vi "Generate Comments.vi"(7 "error in (no error)":errorcluster, 8 "Ring in":refnum<vi>, 9 "cluster":T1) -> (0 "error out":errorcluster, 2 "Comments":string)   [LabVIEW 2016, in "Transport.lvclass"]
uses:
  Transport.lvclass
  Typedefs/Comments-cluster.ctl
  <userlib>/LevyLab/Krohn Hite 7008/typedefs/Gain-Enum.ctl
  <userlib>/LevyLab/Krohn Hite 7008/typedefs/Shunt-Enum.ctl
  <userlib>/LevyLab/Krohn Hite 7008/KH7008.lvclass
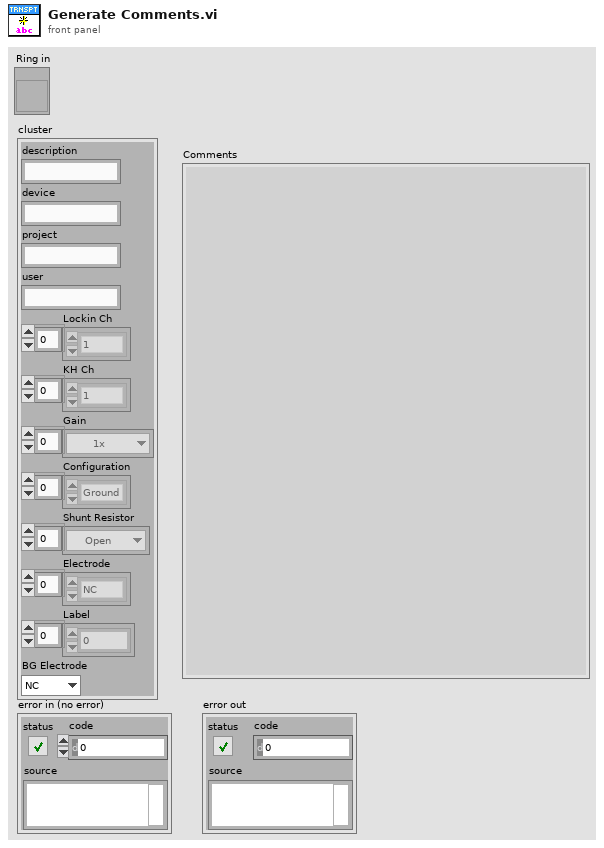
[diagram p1: front panel]
types:
  T1 = typedef "Transport.lvclass/Comments-cluster.ctl" = cluster{"description":string, "device":string, "project":string, "user":string, "Lockin Ch":enum16{"1", "2", "3", "4", "5", "6", "7", "8"}[], "KH Ch":enum16{"1", "2", "3", "4", "5", "6", "7", "8"}[], "Gain":T2[], "Configuration":enum16{"Ground", "Current", "Voltage", "Gate"}[], "Shunt Resistor":T3[], "Electrode":enum16{"NC", "26", "27", "28", "1", "2", "3", "4", "5", "6", "7", "8", "9", "10", "11", "12", "13", "14", "15", "16", "17", "18", "19", "20", "21", "22", "23", "24", "25"}[], "Label":u16[], "BG Electrode":enum16{"NC", "26", "27", "28", "1", "2", "3", "4", "5", "6", "7", "8", "9", "10", "11", "12", "13", "14", "15", "16", "17", "18", "19", "20", "21", "22", "23", "24", "25"}}
  T2 = typedef "KH7008.lvclass/Gain-Enum.ctl" = enum16{"1x", "10x", "100x", "1000x"}
  T3 = typedef "KH7008.lvclass/Shunt-Enum.ctl" = enum16{"Open", "50 Ohms", "500 Ohms", "5k Ohms", "50k Ohms"}
  T4 = enum16{"NC", "26", "27", "28", "1", "2", "3", "4", "5", "6", "7", "8", "9", "10", "11", "12", "13", "14", "15", "16", "17", "18", "19", "20", "21", "22", "23", "24", "25"}[]
  T5 = enum16{"NC", "26", "27", "28", "1", "2", "3", "4", "5", "6", "7", "8", "9", "10", "11", "12", "13", "14", "15", "16", "17", "18", "19", "20", "21", "22", "23", "24", "25"}
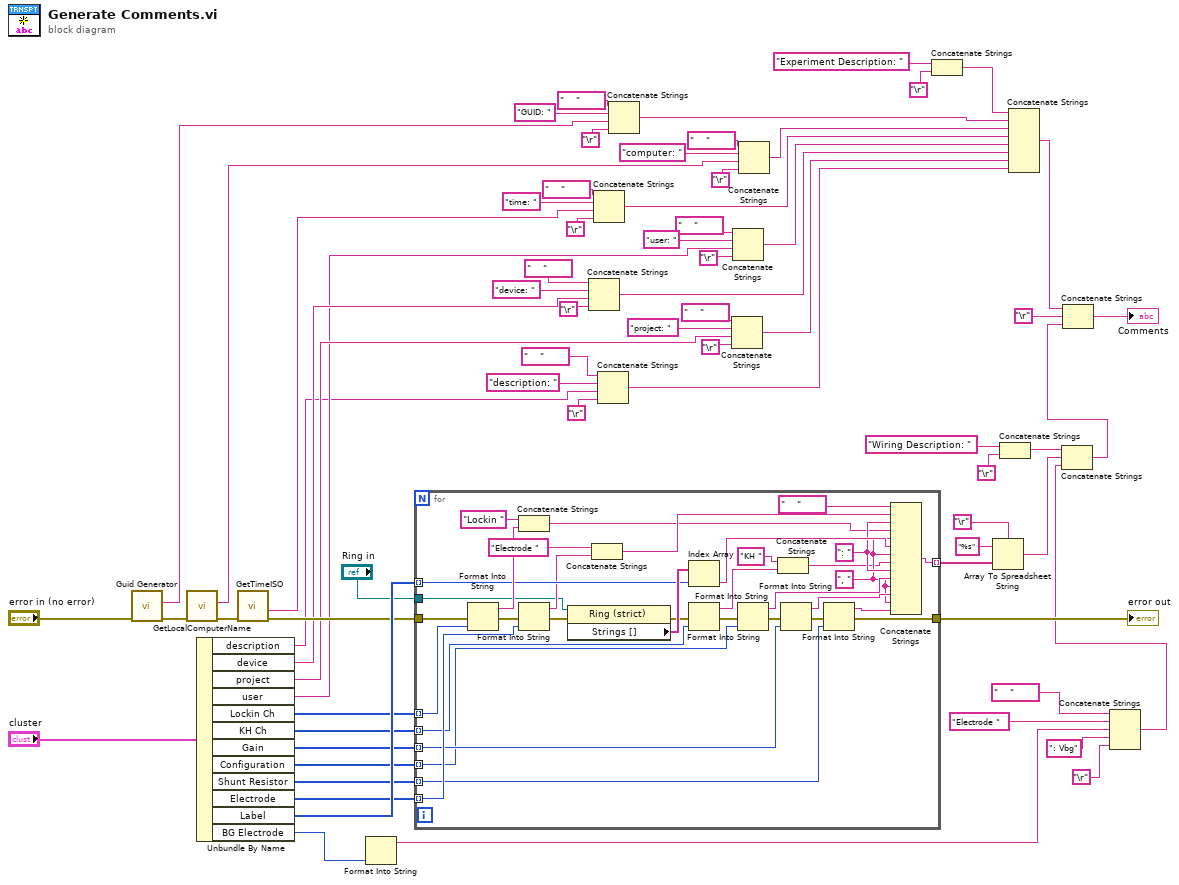
[diagram p0: block diagram]
diagram:
  n1 = call <vilib>:"Guid Generator.vi"("error in (no error)"="error in (no error)") -> ("error out"=w42:errorcluster, "GUID"=w26:string)  [unwired: 9 in]
  n2 = call <userlib>:"GetLocalComputerName.vi"("error in (no error)"=w42) -> ("error out"=w38:errorcluster, "Name"=w22:string)  [unwired: 9 in]
  n3 = Unbundle By Name("cluster") -> ("description"=w40:string, "device"=w50:string, "project"=w49:string, "user"=w48:string, "Lockin Ch"=w64:enum16{"1", "2", "3", "4", "5", "6", "7", "8"}[], "KH Ch"=w65:enum16{"1", "2", "3", "4", "5", "6", "7", "8"}[], "Gain"=w66:T2[], "Configuration"=w67:enum16{"Ground", "Current", "Voltage", "Gate"}[], "Shunt Resistor"=w68:T3[], "Electrode"=w69:T4, "Label"=w70:u16[], "BG Electrode"=w7:T5)
  n4 = call "GetTimeISO.vi"("error in (no error)"=w38) -> ("error out"=w58:errorcluster, "ISO 8601 date-time string"=w41:string)  [unwired: 8 in, 1 out]
  n5 = Format Into String(w7) -> (resulting string=w5:string)  [unwired: 3 in, 1 out]
  n6 = for {
    tunnel: w64 -> [w104] mode=indexing
    tunnel: w65 -> [w83] mode=indexing
    tunnel: w66 -> [w94] mode=indexing
    tunnel: w67 -> [w92] mode=indexing
    tunnel: w68 -> [w87] mode=indexing
    tunnel: w69 -> [w96] mode=indexing
    tunnel: w70 -> [w98] mode=indexing
    tunnel: [w100] -> w59 mode=indexing
    tunnel: "Ring in" -> [w82]
    tunnel: w58 -> [w81]
    tunnel: [w74] -> w57
    w89 = ", "
    w93 = ": "
    n7 = Format Into String(error in=w81, w104) -> (resulting string=w102:string, error out=w80:errorcluster)  [unwired: 2 in]
    n8 = Concatenate Strings("Lockin ", w102) -> (w71:string)
    n9 = Format Into String(error in=w80, w96) -> (resulting string=w95:string, error out=w79:errorcluster)  [unwired: 2 in]
    n10 = property on="Property Node" class="Ring (strict)"(reference=w82, error in=w79) -> (error out=w78:errorcluster, "Strings []"=w99:string[])  [unwired: 1 out]
    n11 = Concatenate Strings("Electrode ", w95) -> (w72:string)
    n12 = Index Array(array=w99, index=w98) -> (element=w97:string)
    n13 = Format Into String(error in=w78, w83) -> (resulting string=w84:string, error out=w77:errorcluster)  [unwired: 2 in]
    n14 = Format Into String(error in=w77, w92) -> (resulting string=w91:string, error out=w76:errorcluster)  [unwired: 2 in]
    n15 = Concatenate Strings("KH ", w84) -> (w85:string)
    n16 = Format Into String(error in=w76, w94) -> (resulting string=w90:string, error out=w75:errorcluster)  [unwired: 2 in]
    n17 = Format Into String(error in=w75, w87) -> (resulting string=w88:string, error out=w74:errorcluster)  [unwired: 2 in]
    n18 = Concatenate Strings("    " ("string"), w72, w93, w71, w89, w97, w89, w85, w93, w91, w89, w90, w89, w88) -> (w100:string)
  }
  "error out" <- w57
  n19 = Concatenate Strings("    " ("string"), "device: " ("string"), w50, "\r") -> (w17:string)
  n20 = Concatenate Strings("    " ("string"), "time: " ("string"), w41, "\r") -> (w19:string)
  n21 = Concatenate Strings("    " ("string"), "description: " ("string"), w40, "\r") -> (w15:string)
  n22 = Concatenate Strings("    " ("string"), "GUID: " ("string"), w26, "\r") -> (w21:string)
  n23 = Concatenate Strings("    " ("string"), "project: " ("string"), w49, "\r") -> (w16:string)
  n24 = Concatenate Strings("    " ("string"), "user: " ("string"), w48, "\r") -> (w18:string)
  n25 = Concatenate Strings("    " ("string"), "computer: " ("string"), w22, "\r") -> (w20:string)
  n26 = Concatenate Strings("Experiment Description: " ("string"), "\r") -> (w30:string)
  n27 = Array To Spreadsheet String(delimiter (Tab)="\r", array=w59, 3:"%s" ("format string")) -> (spreadsheet string=w10:string)
  n28 = Concatenate Strings("Wiring Description: " ("string"), "\r") -> (w11:string)
  n29 = Concatenate Strings(w30, w21, w20, w19, w18, w17, w16, w15) -> (w14:string)
  n30 = Concatenate Strings("    " ("string"), "Electrode ", w5, ": Vbg", "\r") -> (w2:string)
  n31 = Concatenate Strings(w11, w10, w2) -> (w8:string)
  n32 = Concatenate Strings(w14, "\r", w8) -> (→"Comments":string)
